vi "Draw Points Array with Different Radius.vi"(6 "Draw Para":T2={"fill?(F)"=TRUE, "color(black)"=0, "pen"={"Width"=1, "Style"=enum."Solid"}}, 8 "错误输入":errorcluster, 9 "Radius Array":i16[](array[numeric]), 10 "Points Array":T1[](array[typedef]), 11 "Pic in":picture) -> (0 "错误输出":errorcluster, 3 "Pic out":picture)   [LabVIEW 2011, in "Basic Shape.lvlib"]
uses:
  Basic Shape.lvlib
  Draw Para Custom Control.ctl
  Point Custom Control.ctl
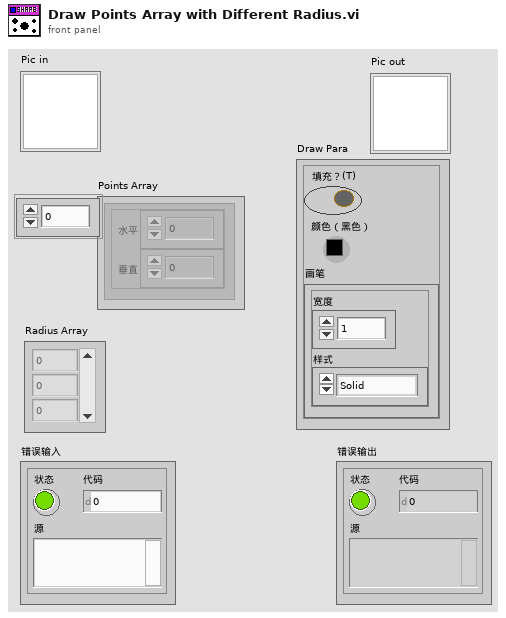
[diagram p1: front panel]
types:
  T1 = typedef "Basic Shape.lvlib/Point Custom Control.ctl" = cluster{"horizontal":i16, "vertical":i16}
  T2 = typedef "Basic Shape.lvlib/Draw Para Custom Control.ctl" = cluster{"fill?(F)":bool, "color(black)":u32, "pen":cluster{"Width":u16, "Style":enum32{"Solid", "Dash", "Dot", "DashDot", "DashDotDot"}}}
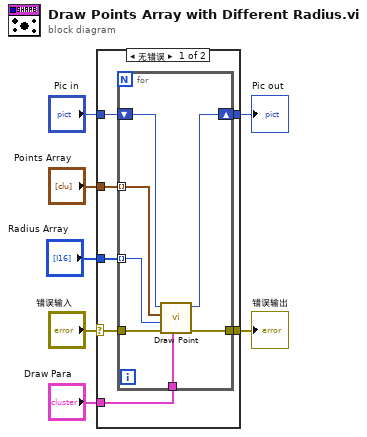
[diagram p0: block diagram]
diagram:
  n1 = case shown="无错误" "错误输入" {
    selector: "错误输入" -> [w9 w23]
    tunnel: [w8 w23] -> w6
    tunnel: "Pic in" -> [w14 w22]
    tunnel: "Draw Para" -> [w10 _]
    tunnel: [w13 w22] -> w3
    tunnel: "Radius Array" -> [w12 _]
    tunnel: "Points Array" -> [w11 _]
    frame No Error {
      n2 = for {
        shift-right: [w20] -> w13
        shift-left: w14 -> [w21]
        tunnel: w12 -> [w19] mode=indexing
        tunnel: w11 -> [w18] mode=indexing
        tunnel: w10 -> [w17]
        tunnel: w9 -> [w16]
        tunnel: [w15] -> w8
        n3 = call "Draw Point.vi"("Draw Para"=w17, "错误输入"=w16, "radius"=w19, "Center"=w18, "Pic in"=w21) -> ("错误输出"=w15:errorcluster, "Pic out"=w20:picture)  [unwired: 5 in]
      }
    }
    frame Error {
    }
  }
  "错误输出" <- w6
  "Pic out" <- w3
